vi "removeDuplicates.vi"(8 "error in (no error)":errorcluster, 9 "Don't add t zero":bool, 10 "times":dbl[](array[numeric]) format="%#_18g", 11 "ScriptEventList in":refnum<class "ScriptEventList.lvclass">) -> (0 "error out":errorcluster, 2 "times out":dbl[](array[numeric]) format="%_10g", 3 "ScriptEventList out":refnum<class "ScriptEventList.lvclass">)   [LabVIEW 2011, in "Tools.lvlib" / "Scripting.lvlib" / "ScriptEventList.lvclass"]
uses:
  ScriptEventList.lvclass
panel:
  out "ceil(x): smallest int >= x":dbl[](array[numeric]) format="%#_10g"
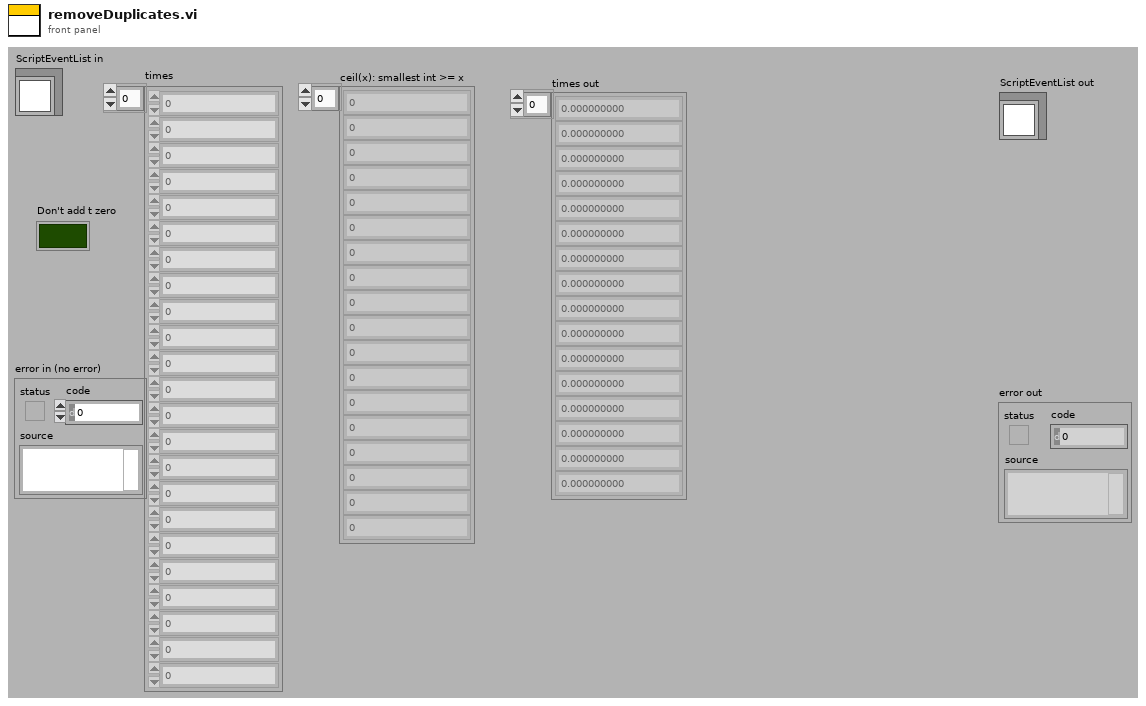
[diagram p1: front panel]
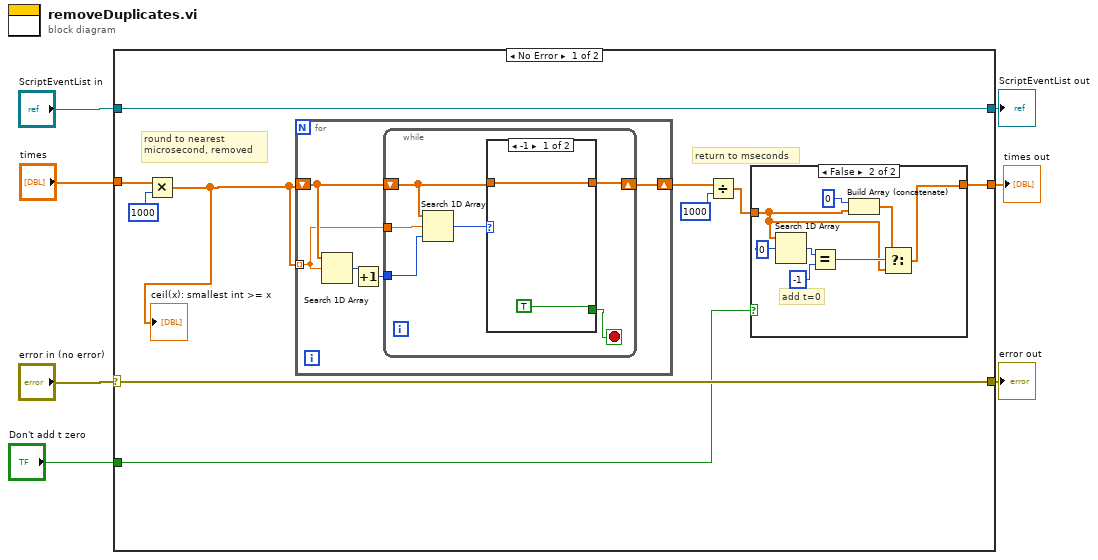
[diagram p0: block diagram]
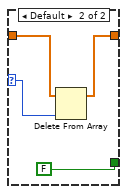
[diagram p3: hidden frame]
diagram:
  n1 = case shown="No Error" "error in (no error)" {
    selector: "error in (no error)" -> [w16 w45]
    tunnel: [w16 w45] -> w6
    tunnel: [w17 w44] -> w4
    tunnel: "ScriptEventList in" -> [w17 w44]
    tunnel: "times" -> [w15 _]
    tunnel: [w10 _] -> w2
    tunnel: "Don't add t zero" -> [w9 _]
    frame No Error {
      # "return to mseconds"
      # "round to nearest\nmicrosecond, removed"
      n2 = Multiply(x=w15, y=1000) -> (x*y=w8:dbl[])
      "ceil(x): smallest int >= x" <- w8
      n3 = for {
        shift-right: [w31] -> w13
        shift-left: w8 -> [w28]
        tunnel: w8 -> [w27] mode=indexing
        n4 = Search 1D Array(1D array=w28, element=w27) -> (index of element=w30:i32)  [unwired: 1 in]
        n5 = Increment(x=w30) -> (x+1=w29:i32)
        n6 = while {
          shift-right: [w35] -> w31
          shift-left: w28 -> [w33]
          tunnel: w29 -> [w34]
          tunnel: w27 -> [w32]
          stop <- w36 stop-if-true
          n7 = Search 1D Array(1D array=w33, element=w32, start index (0)=w34) -> (index of element=w37:i32)
          n8 = case shown="-1" w37 {
            selector: w37 -> [_ w42]
            tunnel: [TRUE FALSE] -> w36
            tunnel: w33 -> [w38 w41]
            tunnel: [w38 w40] -> w35
            frame -1 {
            }
            frame Default {
              n9 = Delete From Array(array=w41, index=w42) -> (array with subset deleted=w40:dbl[])  [unwired: 1 in, 1 out]
            }
          }
        }
      }
      n10 = Divide(x=w13, y=1000) -> (x/y=w11:dbl[])
      n11 = case shown="False" w9 {
        tunnel: w11 -> [w18 w20]
        tunnel: [w18 w19] -> w10
        frame True {
          # "don't add zero\nfor Keithley for example"
        }
        frame False {
          # "add t=0"
          n12 = Search 1D Array(1D array=w20, element=0) -> (index of element=w25:i32)  [unwired: 1 in]
          n13 = Equal?(x=w25, y=-1) -> (x = y?=w23:bool)
          n14 = Build Array (concatenate)(0, w20) -> (w21:dbl[])
          n15 = Select(t=w21, s=w23, f=w20) -> (s? t:f=w19:dbl[])
        }
      }
    }
    frame Error {
    }
  }
  "error out" <- w6
  "ScriptEventList out" <- w4
  "times out" <- w2
